vi "Initialize.vi"(7 "not in use":string="Setpoint.ch%d.SP", 8 "error in":errorcluster, 9 "Number of Channels":u32=1, 10 "Instance Name":string="PluginName", 11 "Temperature Setpoint in":refnum<class "Temperature Setpoint.lvclass">) -> (0 "error out 2":errorcluster, 3 "Temperature Setpoint out":refnum<class "Temperature Setpoint.lvclass">)   [LabVIEW 2023, in "Temperature Setpoint.lvclass"]
uses:
  Temperature Setpoint.lvclass
  Parents/Setpoint/Setpoint.lvclass
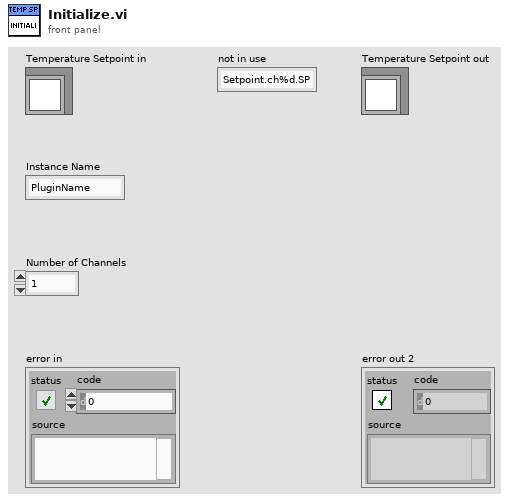
[diagram p1: front panel]
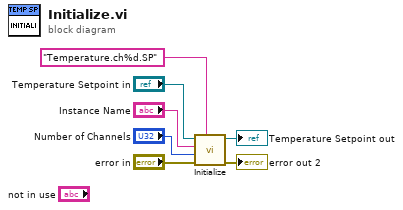
[diagram p0: block diagram]
diagram:
  n1 = call-parent "Initialize.vi"("ChannelName"="Temperature.ch%d.SP", "error in"="error in", "Number of Channels"="Number of Channels", "Instance Name"="Instance Name", "Setpoint in"="Temperature Setpoint in") -> ("error out 2"=→"error out 2":errorcluster, "Setpoint out"=→"Temperature Setpoint out":refnum<class "Temperature Setpoint.lvclass">)  [unwired: 5 in]
